vi "Get Capacity.vi"(1 "Hash Function in":refnum<class "NI_SHA-3.lvclass">) -> (0 "capacity":i32)   [LabVIEW 2020, in "NI_SHA-3.lvclass"]
uses:
  <vilib>/security/Message Digest/SHA-3/NI_SHA-3.lvclass
  <vilib>/security/Message Digest/SHA-3/NI_SHA-3.lvclass/NI_SHA-3.ctl
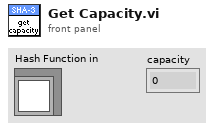
[diagram p1: front panel]
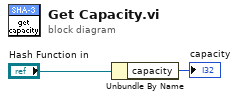
[diagram p0: block diagram]
diagram:
  n1 = Unbundle By Name("Hash Function in") -> ("capacity"=→"capacity":i32)
